vi "Main.vi"() -> ()   [LabVIEW 2020]
uses:
  classes/Folder/Folder.lvclass
  C:/PA_Source/advent-of-code/2022/Paul/07/classes/system object/system object.lvclass
  classes/File/File.lvclass
  <vilib>/regexp/Match Regular Expression.xnode
  classes/system object/system object.lvclass
panel:
  in  "Ready for real?":bool
  out "min value 2":i32
  out "size of file to delate (part b)":i32
  out "needed":i32
  out "sum of folders <= 100k":i32
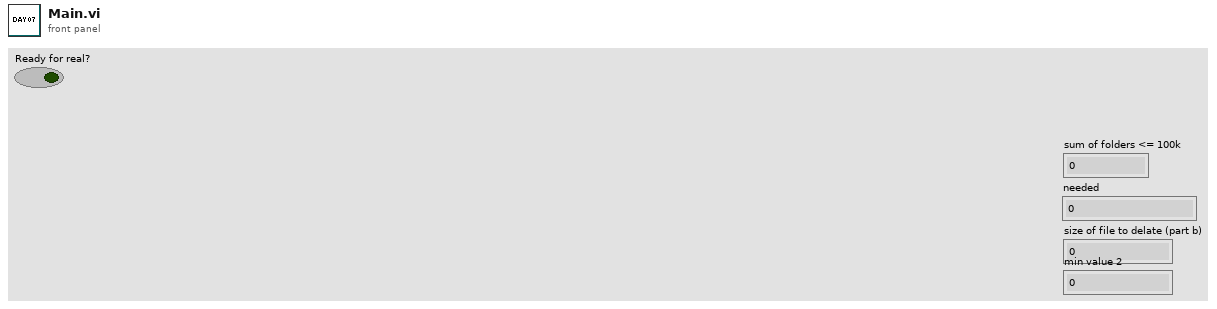
[diagram p1: front panel]
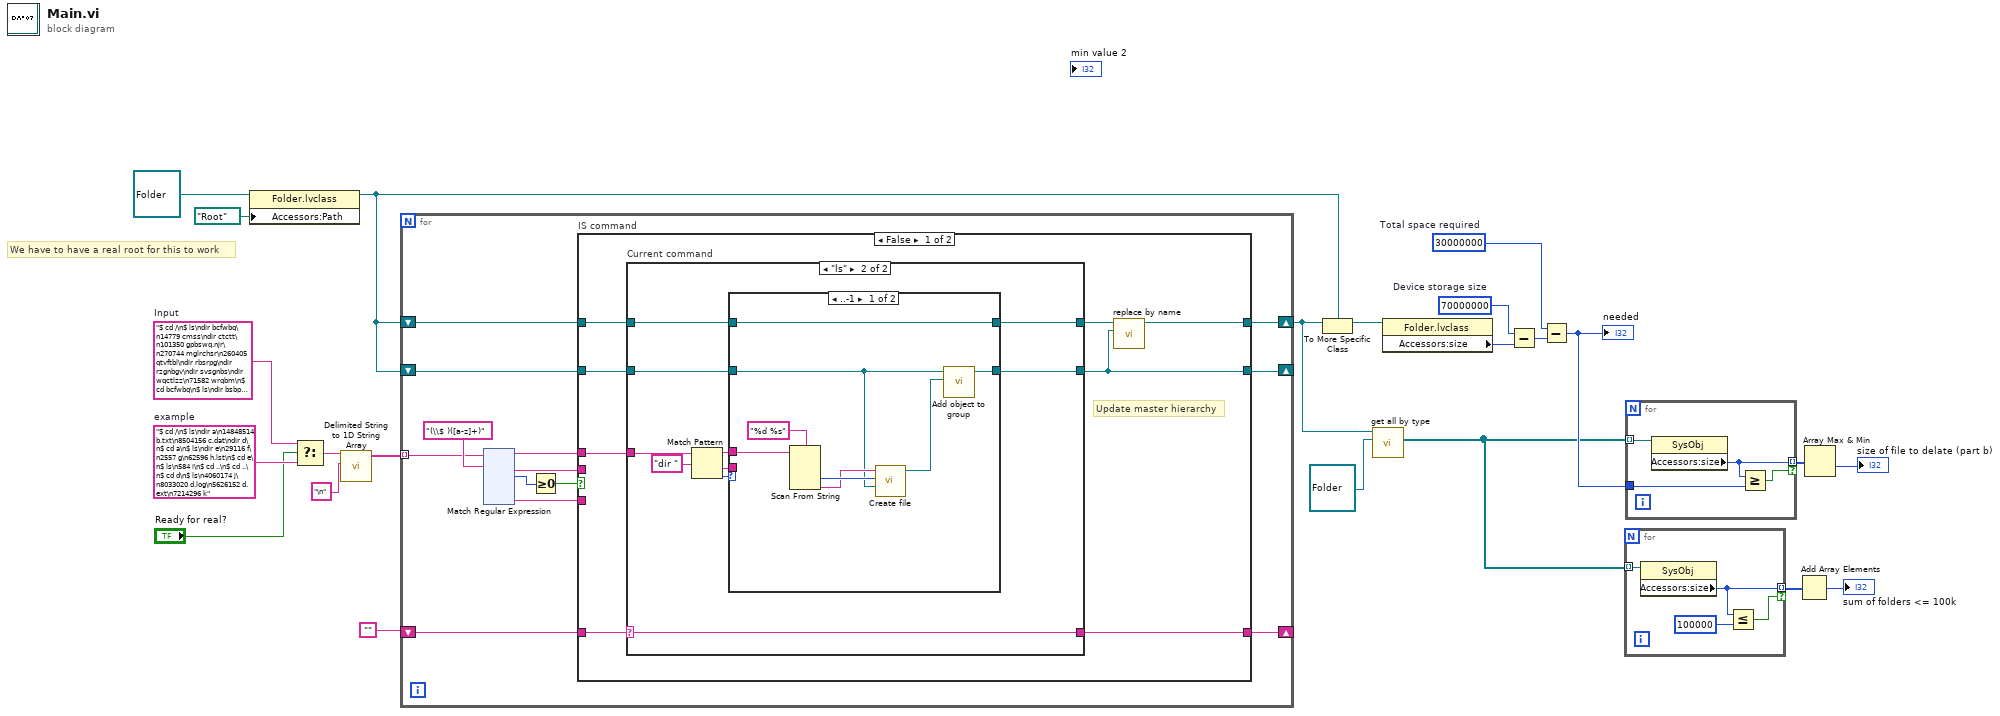
[diagram p0: block diagram]
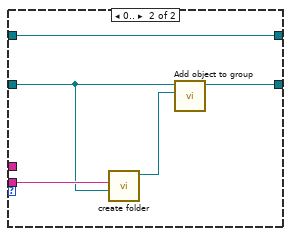
[diagram p3: hidden frame]
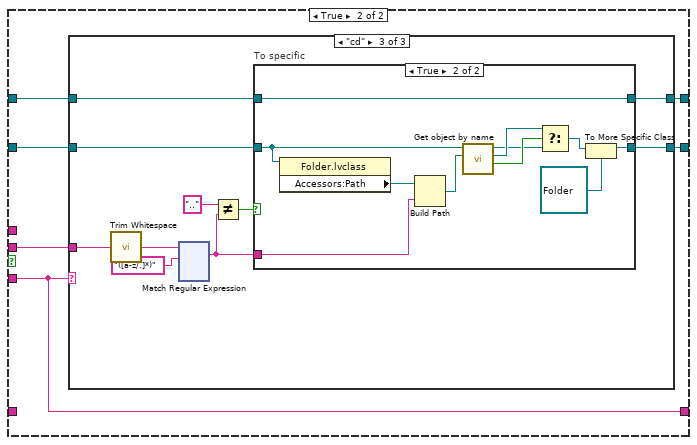
[diagram p4: hidden frame]
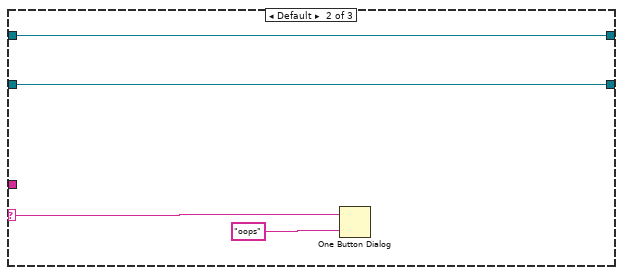
[diagram p6: hidden frame]
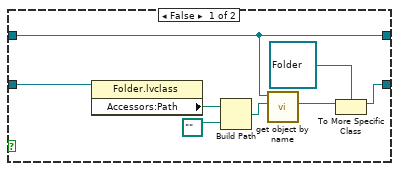
[diagram p7: hidden frame]
diagram:
  w11 = 30000000  # Total space required
  w12 = 70000000  # Device storage size
  w4 = "$ cd /\n$ ls\ndir a\n14848514 b.txt\n8504156 c.dat\ndir d\n$ cd a\n$ ls\ndir e\n29116 f\n2557 g\n62596 h.lst\n$ cd e\n$ ls\n584 i\n$ cd ..\n$ cd ..\n$ cd d\n$ ls\n4060174 j\n8033020 d.log\n5626152 d.ext\n7214296 k"  # example
  w6 = "$ cd /\n$ ls\ndir bcfwbq\n14779 cmss\ndir ctctt\n101350 gpbswq.njr\n270744 mglrchsr\n260405 qtvftbl\ndir rbsrpg\ndir rzgnbgv\ndir svsgnbs\ndir wqctlzz\n71582 wrqbm\n$ cd bcfwbq\n$ ls\ndir bsbpc\ndir gpbswq\n172204 lpn.qjd\n269121 lts.zjd\ndir pfps\ndir phvgmv\ndir pjcrwh\ndir pvf\ndir rthpbmhr\ndir sjnvdz\n$ cd bsbpc\n$ ls\n191305 hlqptq.nrj\n15627 lts.zjd\n$ cd ..\n$ cd gpbswq\n$ ls\ndir ctctt\ndir jcw\ndir jnh\n53143 lts.zjd\ndir qrrjgdbd\ndir tnsjg\n$ cd ctctt\n$ ls\ndir hhmm\n$ cd hhmm\n$ ls\n89761 brfjczv.lmr\n226384 gwqfwwp.ctl\n174778 pgsdmfj\n$ cd ..\n$ cd ..\n$ cd jcw\n$ ls\n149585 gpbswq.lbv\n$ cd ..\n$ cd jnh\n$ ls\n10840 ctctt\ndir fzplg\ndir jvpc\ndir lpn\ndir mcz\n48063 nczc\n8024 rthpbmhr.qwq\n65222 vqgbgm\n$ cd fzplg\n$ ls\n34828 lpn.vcl\ndir svsgnbs\n$ cd svsgnbs\n$ ls\n216427 bvtl\n242012 gpbswq.qlg\ndir gsmltmw\n11388 lpn.trp\ndir lrr\ndir vwqlvj\n$ cd gsmltmw\n$ ls\n66467 pldhhjch\n$ cd ..\n$ cd lrr\n$ ls\ndir ctctt\ndir lpn\n16831 lts.zjd\ndir svsgnbs\ndir tdpmdfgd\n177469 wct.njp\n$ cd ctctt\n$ ls\n145394 phd.tvj\n$ cd ..\n$ cd lpn\n$ ls\ndir svsgnbs\n$ cd svsgnbs\n$ ls\n148504 ctctt.vjd\n$ cd ..\n$ cd ..\n$ cd svsgnbs\n$ ls\n245750 ggbhsgz.snc\n$ cd ..\n$ cd tdpmdfgd\n$ ls\ndir cghfclv\ndir mcfzvlvw\ndir mdgvcgbc\n$ cd cghfclv\n$ ls\n49162 shwslwsf.lww\n$ cd ..\n$ cd mcfzvlvw\n$ ls\ndir bsbswh\n$ cd bsbswh\n$ ls\ndir hqsdsp\n$ cd hqsdsp\n$ ls\n70065 pldhhjch\n$ cd ..\n$ cd ..\n$ cd ..\n$ cd mdgvcgbc\n$ ls\n235514 dhfms.nwl\n$ cd ..\n$ cd ..\n$ cd ..\n$ cd vwqlvj\n$ ls\n269473 jwv.dqh\n90324 mglrchsr\n194977 rwgsvszh.jbf\n$ cd ..\n$ cd ..\n$ cd ..\n$ cd jvpc\n$ ls\ndir rdgqr\ndir sspn\n$ cd rdgqr\n$ ls\ndir qcjccsth\n$ cd qcjccsth\n$ ls\ndir rqwvslc\n$ cd rqwvslc\n$ ls\n275985 pgqph.lcn\n$ cd ..\n$ cd ..\n$ cd ..\n$ cd sspn\n$ ls\n200316 gpbswq\n162820 pldhhjch\n$ cd ..\n$ cd ..\n$ cd lpn\n$ ls\n277995 hlqptq.nrj\n$ cd ..\n$ cd mcz\n$ ls\ndir fjtj\n157693 gqfgrfqw.wtc\ndir jqbpcd\n206235 lpn\n54229 mglrchsr\n238506 rthpbmhr\ndir snr\ndir ztlrtgjl\n$ cd fjtj\n$ ls\n240610 fbwzn\n207688 hlqptq.nrj\n150032 lts.zjd\n48060 mcrgn\n265551 zqrnt.srf\n$ cd ..\n$ cd jqbpcd\n$ ls\n256141 ctctt.nbp\ndir gpbswq\n78480 hmddcjdd.bmc\n31403 lpn\n120619 mvdfjzdr\ndir nqgvl\n$ cd gpbswq\n$ ls\n125791 ctctt\n$ cd ..\n$ cd nqgvl\n$ ls\n174465 jrbfcvf.rqr\n144210 lts.zjd\n258976 rthpbmhr\n$ cd ..\n$ cd ..\n$ cd snr\n$ ls\n185943 rthpbmhr.jhb\n$ cd ..\n$ cd ztlrtgjl\n$ ls\n232309 ntlzfsz.vjd\n254942 zhrds.nbp\n$ cd ..\n$ cd ..\n$ cd ..\n$ cd qrrjgdbd\n$ ls\ndir gpbswq\n$ cd gpbswq\n$ ls\n170768 rthpbmhr.qwf\n$ cd ..\n$ cd ..\n$ cd tnsjg\n$ ls\n242206 bjmgvmp.hht\n245356 frtdp\ndir jrflhz\n128115 lpn\n120081 rfhs\ndir sfplvt\ndir tts\n114165 zfl.ccr\n$ cd jrflhz\n$ ls\ndir gpbswq\ndir nnlzjwts\ndir sctf\n$ cd gpbswq\n$ ls\n121401 mglrchsr\n$ cd ..\n$ cd nnlzjwts\n$ ls\ndir gljnss\n165011 lts.zjd\n69364 svsgnbs.bqm\n$ cd gljnss\n$ ls\n181850 cfjbd.fmj\n$ cd ..\n$ cd ..\n$ cd sctf\n$ ls\n109435 gqfgrfqw.wtc\n146343 lpn.mbs\n255948 svsgnbs.hbf\n231472 vdrfwqwv.pzf\n263352 zgzj\n$ cd ..\n$ cd ..\n$ cd sfplvt\n$ ls\n51580 hlqptq.nrj\ndir mldph\n$ cd mldph\n$ ls\n163815 hsnw\n$ cd ..\n$ cd ..\n$ cd tts\n$ ls\ndir ctctt\n211239 rpm\ndir rthpbmhr\ndir wpnnrzb\n$ cd ctctt\n$ ls\ndir ctctt\n137333 hshpfwl\n183146 srd\n$ cd ctctt\n$ ls\n89470 hlqptq.nrj\n$ cd ..\n$ cd ..\n$ cd rthpbmhr\n$ ls\n139569 fhjlbrmp.phd\n223589 jvrs.bpj\n198566 rthpbmhr.qdr\n$ cd ..\n$ cd wpnnrzb\n$ ls\ndir ctctt\n158058 fjtcc\ndir jqqhgjv\ndir qvbvvb\n16429 wds.hpj\n$ cd ctctt\n$ ls\n166551 gcjt.wld\n233189 gpbswq.mls\n193694 rthpbmhr.rvz\ndir svsgnbs\n$ cd svsgnbs\n$ ls\n248185 fpssfvd.zft\n215781 rwtg.gch\n$ cd ..\n$ cd ..\n$ cd jqqhgjv\n$ ls\ndir gpbswq\n14842 lts.zjd\ndir mqp\n258342 pldhhjch\n103492 sddj.sbq\n248024 svsgnbs\n$ cd gpbswq\n$ ls\ndir sqchbqc\n176209 vdq.jbz\n$ cd sqchbqc\n$ ls\ndir cphf\n$ cd cphf\n$ ls\n253613 snzbgfs.rjf\n$ cd ..\n$ cd ..\n$ cd ..\n$ cd mqp\n$ ls\n10090 mfw\n$ cd ..\n$ cd ..\n$ cd qvbvvb\n$ ls\ndir mzw\ndir svsgnbs\n$ cd mzw\n$ ls\n98994 mmv.hcl\n$ cd ..\n$ cd svsgnbs\n$ ls\n108748 lts.zjd\n10351 mglrchsr\n$ cd ..\n$ cd ..\n$ cd ..\n$ cd ..\n$ cd ..\n$ cd ..\n$ cd pfps\n$ ls\ndir cpp\n110535 mglrchsr\n120669 qvh.fbm\n$ cd cpp\n$ ls\ndir htnmrjpq\n$ cd htnmrjpq\n$ ls\n120225 bdjmsbg.wfz\n$ cd ..\n$ cd ..\n$ cd ..\n$ cd phvgmv\n$ ls\n113550 pldhhjch\n31171 zcfm\n$ cd ..\n$ cd pjcrwh\n$ ls\n265625 snbjdmg.jtn\n$ cd ..\n$ cd pvf\n$ ls\n91010 ctctt\ndir hdz\ndir qtwfpmvz\n$ cd hdz\n$ ls\n103787 rlnrs\n$ cd ..\n$ cd qtwfpmvz\n$ ls\n244905 lts.zjd\n$ cd ..\n$ cd ..\n$ cd rthpbmhr\n$ ls\ndir phq\ndir svsgnbs\ndir wzwfz\ndir zpwfj\n$ cd phq\n$ ls\n91709 bzfnqh\ndir ccwqrjn\ndir gpbswq\ndir svsgnbs\n$ cd ccwqrjn\n$ ls\n8953 fffqzmqp\ndir ftnb\ndir svsgnbs\n$ cd ftnb\n$ ls\n226615 rthpbmhr\n$ cd ..\n$ cd svsgnbs\n$ ls\ndir bhnnm\ndir tjrqtmd\n$ cd bhnnm\n$ ls\ndir prfqw\n$ cd prfqw\n$ ls\ndir hzsjlq\n$ cd hzsjlq\n$ ls\n99285 cfpwbvp\n$ cd ..\n$ cd ..\n$ cd ..\n$ cd tjrqtmd\n$ ls\n237461 cqr.wfj\n149955 zchnb\n$ cd ..\n$ cd ..\n$ cd ..\n$ cd gpbswq\n$ ls\ndir bqqtnfb\ndir ctctt\n261108 gpbswq\n135193 hnrflng\n264503 jrp.bls\n224864 mghhgrj.tgp\ndir pljbtbn\ndir rthpbmhr\n244222 svsgnbs.rzp\n$ cd bqqtnfb\n$ ls\ndir jnzfr\n$ cd jnzfr\n$ ls\ndir bdrqmr\n168907 pldhhjch\n$ cd bdrqmr\n$ ls\n151767 vfw.jjc\n$ cd ..\n$ cd ..\n$ cd ..\n$ cd ctctt\n$ ls\ndir zdsshmr\n$ cd zdsshmr\n$ ls\n77208 hlqptq.nrj\n$ cd ..\n$ cd ..\n$ cd pljbtbn\n$ ls\n63719 hlqptq.nrj\n103719 jjctg.dhw\n547 tljz.wnv\n$ cd ..\n$ cd rthpbmhr\n$ ls\ndir sjbfhcpc\n$ cd sjbfhcpc\n$ ls\n184946 sgpgszw\n$ cd ..\n$ cd ..\n$ cd ..\n$ cd svsgnbs\n$ ls\ndir ctctt\ndir flzsvb\ndir pbw\n23408 qprlnvwv.jmz\ndir wjhplc\n$ cd ctctt\n$ ls\n11507 cnf\ndir gpbswq\n87778 rthpbmhr.wzv\ndir slmbb\ndir sqc\n75556 wsbzwn.mpf\n$ cd gpbswq\n$ ls\n173498 dsg\n202811 msvs.szd\n208419 pldhhjch\n$ cd ..\n$ cd slmbb\n$ ls\ndir jcth\ndir njldhbln\n$ cd jcth\n$ ls\n6106 hlqptq.nrj\n$ cd ..\n$ cd njldhbln\n$ ls\n241153 mvnvzqfc.rtn\n$ cd ..\n$ cd ..\n$ cd sqc\n$ ls\ndir zhrc\n$ cd zhrc\n$ ls\ndir qswqqzb\n$ cd qswqqzb\n$ ls\n264937 btqmqn.hqv\n$ cd ..\n$ cd ..\n$ cd ..\n$ cd ..\n$ cd flzsvb\n$ ls\n58735 hlqptq.nrj\n$ cd ..\n$ cd pbw\n$ ls\n80787 bgfmdg\n234807 gqfgrfqw.wtc\n44816 pldhhjch\ndir qjjpmq\ndir rthpbmhr\n153500 ssmdz\n$ cd qjjpmq\n$ ls\n155209 ctghhsdh\n182544 fprdp.ffs\n$ cd ..\n$ cd rthpbmhr\n$ ls\n136673 lts.zjd\n$ cd ..\n$ cd ..\n$ cd wjhplc\n$ ls\n246593 hhcgnfjb.nbl\n29266 hlqptq.nrj\n246096 lts.zjd\n40242 rrfgvvhg\n$ cd ..\n$ cd ..\n$ cd ..\n$ cd svsgnbs\n$ ls\n215743 fwm\n236816 gqfgrfqw.wtc\n235185 sjdlr.rzj\ndir ztsgb\n$ cd ztsgb\n$ ls\n265998 rthpbmhr.pdp\n275979 zqfcprz.wtd\n$ cd ..\n$ cd ..\n$ cd wzwfz\n$ ls\ndir bsqwtf\ndir ctctt\ndir lpng\ndir svsgnbs\n$ cd bsqwtf\n$ ls\ndir rhjb\ndir sgzvb\n$ cd rhjb\n$ ls\n166599 rthpbmhr.msg\n$ cd ..\n$ cd sgzvb\n$ ls\n185594 zmnb.bcq\n$ cd ..\n$ cd ..\n$ cd ctctt\n$ ls\n130367 svsgnbs\n17459 tdsztr.fsn\n242273 wfs\n$ cd ..\n$ cd lpng\n$ ls\n145778 snmcwfg.hjz\n$ cd ..\n$ cd svsgnbs\n$ ls\ndir ctctt\ndir nqrlzg\ndir qczmdfm\n54814 wtmjh.jdv\n$ cd ctctt\n$ ls\n244171 pldhhjch\n$ cd ..\n$ cd nqrlzg\n$ ls\ndir qjhlj\n$ cd qjhlj\n$ ls\ndir gncct\n$ cd gncct\n$ ls\n141943 wsdgmdd.ctz\n$ cd ..\n$ cd ..\n$ cd ..\n$ cd qczmdfm\n$ ls\n4482 lpn.fmp\n$ cd ..\n$ cd ..\n$ cd ..\n$ cd zpwfj\n$ ls\n226995 lts.zjd\ndir sflcgdm\n$ cd sflcgdm\n$ ls\n199168 bjrjrrm.bfw\ndir fpcq\n24906 gdzfmhz.jhp\n7267 hdpzvh.ngg\ndir jjsgqb\n137796 psws.hvp\n$ cd fpcq\n$ ls\n195792 nghcc.wps\n$ cd ..\n$ cd jjsgqb\n$ ls\n18774 ctctt\n106399 jvbgfhs\n208035 rthpbmhr\ndir zptz\n$ cd zptz\n$ ls\n278792 gqfgrfqw.wtc\n$ cd ..\n$ cd ..\n$ cd ..\n$ cd ..\n$ cd ..\n$ cd sjnvdz\n$ ls\ndir fchgggp\ndir gldg\n40164 gnh.gmv\ndir lpn\ndir njtgjt\n81415 qqfm.grb\ndir vvcbjct\n$ cd fchgggp\n$ ls\ndir fjcclj\ndir lpn\n145291 lts.zjd\n7288 mglrchsr\ndir pmhdzvfn\ndir qtpdfwh\ndir vjwtvb\n$ cd fjcclj\n$ ls\n28333 gpbswq.vtg\n258676 lts.zjd\n$ cd ..\n$ cd lpn\n$ ls\n197797 pldhhjch\n$ cd ..\n$ cd pmhdzvfn\n$ ls\n21538 gpbswq.pwq\n5451 hqjg\ndir llhp\n220717 lzqmh.stl\n123800 pldhhjch\ndir pmv\ndir rzs\ndir tztv\n160018 zfvgjtzr.qth\n$ cd llhp\n$ ls\ndir lsft\ndir pfjmphs\n$ cd lsft\n$ ls\n78424 gpbswq.ddb\n101497 gqfgrfqw.wtc\n137686 hlqptq.nrj\n122325 mglrchsr\n$ cd ..\n$ cd pfjmphs\n$ ls\n185141 mbw.gnd\n$ cd ..\n$ cd ..\n$ cd pmv\n$ ls\n139255 gqfgrfqw.wtc\n272882 hlqptq.nrj\n$ cd ..\n$ cd rzs\n$ ls\ndir gpbswq\n89153 gpbswq.vcv\n81882 gqfgrfqw.wtc\n39252 hlqptq.nrj\ndir tmcm\n$ cd gpbswq\n$ ls\n205674 ctctt.gqd\n$ cd ..\n$ cd tmcm\n$ ls\n156591 gmjvzj.wzl\n199254 lts.zjd\ndir vzhbsdd\ndir zfs\n$ cd vzhbsdd\n$ ls\n70059 gsgzqgn.fhf\n43456 hrttvrqc\n$ cd ..\n$ cd zfs\n$ ls\n223726 hlqptq.nrj\n$ cd ..\n$ cd ..\n$ cd ..\n$ cd tztv\n$ ls\n200126 lpn.bns\ndir wfjwmbj\n$ cd wfjwmbj\n$ ls\n120344 gdqgml.gdn\n$ cd ..\n$ cd ..\n$ cd ..\n$ cd qtpdfwh\n$ ls\ndir qszjt\n$ cd qszjt\n$ ls\n7207 rthpbmhr.rpv\n20452 ztdnfmgp.dsb\n$ cd ..\n$ cd ..\n$ cd vjwtvb\n$ ls\ndir scswlmn\n$ cd scswlmn\n$ ls\n207195 svsgnbs.jqq\n$ cd ..\n$ cd ..\n$ cd ..\n$ cd gldg\n$ ls\n119560 ctctt.wbc\n203041 gqfgrfqw.wtc\ndir hrp\n274270 lts.zjd\n25081 mhsfdhjr.ndw\ndir svsgnbs\n$ cd hrp\n$ ls\ndir lpn\n$ cd lpn\n$ ls\ndir gpbswq\ndir wvrzhdb\n$ cd gpbswq\n$ ls\ndir vtgc\n$ cd vtgc\n$ ls\n231107 hlqptq.nrj\n$ cd ..\n$ cd ..\n$ cd wvrzhdb\n$ ls\n83303 lts.zjd\n$ cd ..\n$ cd ..\n$ cd ..\n$ cd svsgnbs\n$ ls\ndir fhfqlv\n13446 frn.hzg\n126475 wmjjjl.cjr\n$ cd fhfqlv\n$ ls\n243574 hjn.jzb\n$ cd ..\n$ cd ..\n$ cd ..\n$ cd lpn\n$ ls\ndir mqglznd\n$ cd mqglznd\n$ ls\ndir gpbswq\n177654 gpbswq.zhv\n128217 gqfgrfqw.wtc\n66750 hlqptq.nrj\n136018 hvphz\ndir pswvwtf\n113363 rthpbmhr.gwz\ndir twddrn\n$ cd gpbswq\n$ ls\n244278 lts.zjd\ndir pfrjwbvl\ndir qlrfw\n222491 rthpbmhr\n$ cd pfrjwbvl\n$ ls\n46802 cfl.ljt\ndir ctctt\ndir dfqzmd\n110525 gshdhsfm\ndir jcbw\ndir lpn\n237385 pldhhjch\n15812 prcwhhq.jjh\ndir rthpbmhr\n260693 zmgq\n$ cd ctctt\n$ ls\n6529 hctcg.dpw\n188655 lpn.qjf\n202221 wjnb\n$ cd ..\n$ cd dfqzmd\n$ ls\n197980 ctctt\n$ cd ..\n$ cd jcbw\n$ ls\n1281 gpbswq\n15778 jfgjlcd.mqh\n38803 mdtcrb.dbj\ndir qtjbpbs\n$ cd qtjbpbs\n$ ls\n59348 mglrchsr\n$ cd ..\n$ cd ..\n$ cd lpn\n$ ls\ndir ctctt\ndir hsjjp\n260465 mglrchsr\n$ cd ctctt\n$ ls\ndir wvbrsb\n$ cd wvbrsb\n$ ls\n135584 lts.zjd\n$ cd ..\n$ cd ..\n$ cd hsjjp\n$ ls\n249448 ddfqnwgf\n164051 dsnhsbp.wvv\ndir fmzgm\ndir gpbswq\n113907 gqfgrfqw.wtc\n$ cd fmzgm\n$ ls\n150025 ngnqjcj.tbf\n$ cd ..\n$ cd gpbswq\n$ ls\n33139 dmgqhf.nzd\ndir gpbswq\ndir rwd\n$ cd gpbswq\n$ ls\n148820 lnqqds.rpg\n$ cd ..\n$ cd rwd\n$ ls\n133433 pldhhjch\n$ cd ..\n$ cd ..\n$ cd ..\n$ cd ..\n$ cd rthpbmhr\n$ ls\n262342 fdnr.svq\ndir nbpsdm\n161791 pldhhjch\n6835 qvclr\n228110 whf\n$ cd nbpsdm\n$ ls\ndir rthpbmhr\ndir svsgnbs\n$ cd rthpbmhr\n$ ls\n267109 chb\n$ cd ..\n$ cd svsgnbs\n$ ls\n150446 rlv.vcc\n$ cd ..\n$ cd ..\n$ cd ..\n$ cd ..\n$ cd qlrfw\n$ ls\ndir sgcpwst\n$ cd sgcpwst\n$ ls\ndir fss\n$ cd fss\n$ ls\n244165 gpbswq.qtz\n$ cd ..\n$ cd ..\n$ cd ..\n$ cd ..\n$ cd pswvwtf\n$ ls\n162099 jhdrnv.zrd\n54856 mglrchsr\ndir psdz\n169053 qhq\n$ cd psdz\n$ ls\ndir lbcf\n$ cd lbcf\n$ ls\n218770 ctctt.chv\n95266 pldhhjch\n$ cd ..\n$ cd ..\n$ cd ..\n$ cd twddrn\n$ ls\n120791 hlqptq.nrj\n212213 vffj\n$ cd ..\n$ cd ..\n$ cd ..\n$ cd njtgjt\n$ ls\ndir mzwdb\n$ cd mzwdb\n$ ls\n108520 lts.zjd\n$ cd ..\n$ cd ..\n$ cd vvcbjct\n$ ls\n155890 ctctt.fbw\n$ cd ..\n$ cd ..\n$ cd ..\n$ cd ctctt\n$ ls\n5656 mpftwp.nds\n8998 pldhhjch\n185601 snrng.qsv\n$ cd ..\n$ cd rbsrpg\n$ ls\n113129 cpwmjw.rbj\ndir jdhmlzr\n114254 sqj.fzp\n120708 svsgnbs.hpn\n$ cd jdhmlzr\n$ ls\ndir cdnmflmm\n248055 hlqptq.nrj\n247942 pldhhjch\ndir qrwsnzdv\n80053 svsgnbs\n219309 zhqgvd.bhw\n$ cd cdnmflmm\n$ ls\n83138 lpn.wtg\n$ cd ..\n$ cd qrwsnzdv\n$ ls\n197145 zspfb.sbd\n$ cd ..\n$ cd ..\n$ cd ..\n$ cd rzgnbgv\n$ ls\n208692 clz\ndir tmcqcpfc\ndir twlnjr\n$ cd tmcqcpfc\n$ ls\ndir jtnf\n$ cd jtnf\n$ ls\n242978 fhvtvdff.swr\n21748 lwcplzmw\n$ cd ..\n$ cd ..\n$ cd twlnjr\n$ ls\ndir ctctt\ndir gpbswq\n98435 rthpbmhr.pcr\ndir snpm\ndir svsgnbs\n104969 zzd\n$ cd ctctt\n$ ls\n200382 pqswsnhp\n$ cd ..\n$ cd gpbswq\n$ ls\n90380 qqrfbwn\n$ cd ..\n$ cd snpm\n$ ls\n57996 swfjlfh.qft\n$ cd ..\n$ cd svsgnbs\n$ ls\n86028 clcfrnr.jwl\n199666 ctctt.ftr\n200949 ctctt.mrh\n23594 dhlmbh.gjt\n278047 mbchg\ndir pgfhp\n$ cd pgfhp\n$ ls\n21555 rlblnvsd\n$ cd ..\n$ cd ..\n$ cd ..\n$ cd ..\n$ cd svsgnbs\n$ ls\n155183 jgjj.sgs\n28150 pldhhjch\n$ cd ..\n$ cd wqctlzz\n$ ls\n23662 mglrchsr\n60923 pldhhjch"  # Input
  # "We have to have a real root for this to work"
  n1 = property class="Folder.lvclass"(reference=refnum<class "Folder.lvclass"> refnum ("Folder.lvclass 2"), "Accessors:Path"=path "/Root" ("Path")) -> (reference out=w18:refnum<class "Folder.lvclass">)  [unwired: 1 in, 1 out]
  n2 = Select(t=w6, s="Ready for real?", f=w4) -> (s? t:f=w5:string)
  n3 = call <vilib>:"Delimited String to 1D String Array.vi"("delimiter"="\n", "delimited string"=w5) -> ("string array"=w22:string[])  [unwired: 9 in]
  n4 = for {
    tunnel: w22 -> [w28] mode=indexing
    shift-right: [w33] -> w19
    shift-left: w18 -> [w34]
    shift-right: [w27] -> _
    shift-left: w18 -> [w32]
    shift-right: [w31] -> _
    shift-left: "" -> [w30]
    n5 = xnode "Match Regular Expression"("input string"=w28, "regular expression"="(\\$ )([a-z]+)") -> ("before match"=w29:string, "after match"=w26:string, "offset past match"=w35:i32, "submatch 2"=w25:string)  [unwired: 4 in, 3 out]
    n6 = Greater Or Equal To 0?(x=w35) -> (x >= 0?=w24:bool)
    n7 = case "IS command" shown="False" w24 {
      tunnel: w34 -> [w158 w193]
      tunnel: [w155 w192] -> w33
      tunnel: [w154 w191] -> w27
      tunnel: w32 -> [w159 w190]
      tunnel: [w157 w189] -> w31
      tunnel: w30 -> [w161 _]
      tunnel: w29 -> [w160 _]
      tunnel: w26 -> [_ w188]
      tunnel: w25 -> [_ w189]
      frame False {
        # "Update master hierarchy"
        n8 = case "Current command" shown="\"ls\"" w161 {
          selector: w161 -> [w162 w167]
          tunnel: w160 -> [_ w174]
          tunnel: w159 -> [w164 w169]
          tunnel: [w164 w165] -> w154
          tunnel: w158 -> [w163 w168]
          tunnel: [w163 w166] -> w156
          tunnel: [w162 w167] -> w157
          frame "False", Default {
          }
          frame "ls" {
            n9 = Match Pattern(string=w174, regular expression="dir ") -> (before substring=w172:string, after substring=w170:string, offset past match=w173:i32)  [unwired: 1 in, 1 out]
            n10 = case shown="..-1" w173 {
              tunnel: w172 -> [w182 _]
              tunnel: w170 -> [_ w187]
              tunnel: w169 -> [w175 w183]
              tunnel: [w177 w185] -> w165
              tunnel: w168 -> [w176 w184]
              tunnel: [w176 w184] -> w166
              frame ..-1 {
                n11 = Scan From String(format string="%d %s", input string=w182) -> (output 1=w180:i32, output 2=w179:string)  [unwired: 4 in, 3 out]
                n12 = call "Create file.vi"("Parent"=w175, "size"=w180, "name"=w179) -> ("File out"=w178:refnum<class "File.lvclass">)  [unwired: 7 in, 1 out]
                n13 = call-dynamic "Add object to group.vi"("system object"=w178, "Folder in"=w175) -> ("Folder out"=w177:refnum<class "Folder.lvclass">)  [unwired: 8 in, 1 out]
              }
              frame 0.. {
                n14 = call "create folder.vi"("Parent"=w183, "name"=w187) -> ("Folder.lvclass"=w186:refnum<class "Folder.lvclass">)  [unwired: 9 in]
                n15 = call-dynamic "Add object to group.vi"("system object"=w186, "Folder in"=w183) -> ("Folder out"=w185:refnum<class "Folder.lvclass">)  [unwired: 8 in, 1 out]
              }
            }
          }
        }
        n16 = call-dynamic "replace by name.vi"("New object"=w154, "SysObj in"=w156) -> ("SysObj out"=w155:refnum<class "system object.lvclass">)  [unwired: 7 in, 2 out]
      }
      frame True {
        n17 = case shown="\"cd\"" w189 {
          selector: w189 -> [_ w199 _]
          tunnel: w193 -> [w195 w197 w209]
          tunnel: [w195 w197 w207] -> w192
          tunnel: [w194 w196 w206] -> w191
          tunnel: w190 -> [w194 w196 w208]
          tunnel: w188 -> [_ _ w204]
          frame "ls" {
          }
          frame Default {
            n18 = One Button Dialog(message=w199, button name ("OK")="oops") -> ()  [unwired: 1 out]
          }
          frame "cd" {
            n19 = call <vilib>:"Trim Whitespace.vi"("string"=w204) -> ("trimmed string"=w205:string)  [unwired: 1 in]
            n20 = xnode "Match Regular Expression"("input string"=w205, "regular expression"="([a-z/.]*)") -> ("whole match"=w200:string)  [unwired: 4 in, 4 out]
            n21 = Not Equal?(x="..", y=w200) -> (x != y?=w201:bool)
            n22 = case "To specific" shown="True" w201 {
              tunnel: w208 -> [w331 w335]
              tunnel: [w328 w338] -> w206
              tunnel: w209 -> [w327 w336]
              tunnel: [w327 w336] -> w207
              tunnel: w200 -> [_ w332]
              frame False {
                n23 = property class="Folder.lvclass"(reference=w331) -> ("Accessors:Path"=w325:path)  [unwired: 1 in, 2 out]
                n24 = Build Path(base path=w325, name or relative path=path "..") -> (appended path=w326:path)
                n25 = call-dynamic "get object by name.vi"("Name"=w326, "system object in"=w327) -> ("Target object"=w330:refnum<class "system object.lvclass">)  [unwired: 6 in, 3 out]
                n26 = To More Specific Class(target class=refnum<class "Folder.lvclass"> refnum ("Folder.lvclass"), reference=w330) -> (specific class reference=w328:refnum<class "Folder.lvclass">)  [unwired: 1 in, 1 out]
              }
              frame True {
                n27 = property class="Folder.lvclass"(reference=w335) -> ("Accessors:Path"=w334:path)  [unwired: 1 in, 2 out]
                n28 = Build Path(base path=w334, name or relative path=w332) -> (appended path=w333:path)
                n29 = call-dynamic "Get object by name.vi"("path"=w333, "Folder in"=w335) -> ("Found"=w342:bool, "Object"=w341:refnum<class "system object.lvclass">, "Folder out"=w340:refnum<class "Folder.lvclass">)  [unwired: 6 in, 1 out]
                n30 = Select(t=w341, s=w342, f=w340) -> (s? t:f=w339:refnum<class "system object.lvclass">)
                n31 = To More Specific Class(target class=refnum<class "Folder.lvclass"> refnum ("Folder.lvclass"), reference=w339) -> (specific class reference=w338:refnum<class "Folder.lvclass">)  [unwired: 1 in, 1 out]
              }
            }
          }
        }
      }
    }
  }
  n32 = To More Specific Class(target class=w18, reference=w19) -> (specific class reference=w15:refnum<class "Folder.lvclass">)  [unwired: 1 in, 1 out]
  n33 = call-dynamic "get all by type.vi"("Type"=refnum<class "Folder.lvclass"> refnum ("Folder.lvclass"), "SysObj in"=w19) -> ("All objects"=w9:refnum<class "system object.lvclass">[])  [unwired: 7 in, 2 out]
  n34 = property class="Folder.lvclass"(reference=w15) -> ("Accessors:size"=w14:i32)  [unwired: 1 in, 2 out]
  n35 = Subtract(x=w12, y=w14) -> (x-y=w13:i32)
  n36 = Subtract(x=w11, y=w13) -> (x-y=w10:i32)
  "needed" <- w10
  n37 = for {
    tunnel: w9 -> [w346] mode=indexing
    tunnel: [w345] -> w17 mode=indexing if=w344
    n38 = property class="SysObj"(reference=w346) -> ("Accessors:size"=w345:i32)  [unwired: 1 in, 2 out]
    n39 = Less Or Equal?(x=w345, y=100000) -> (x <= y?=w344:bool)
  }
  n40 = for {
    tunnel: w9 -> [w350] mode=indexing
    tunnel: [w349] -> w8 mode=indexing if=w347
    tunnel: w10 -> [w348]
    n41 = property class="SysObj"(reference=w350) -> ("Accessors:size"=w349:i32)  [unwired: 1 in, 2 out]
    n42 = Greater Or Equal?(x=w349, y=w348) -> (x >= y?=w347:bool)
  }
  n43 = Add Array Elements(numeric array=w17) -> (sum=→"sum of folders <= 100k":i32)
  n44 = Array Max & Min(array=w8) -> (min value=→"size of file to delate (part b)":i32)  [unwired: 3 out]
